vi "moc_energia_sygn_okr.vi"() -> ()   [LabVIEW 2025]
uses:
  <vilib>/measure/NI_MABase.lvlib
panel:
  out "gestosc widmowa mocy":waveform(dbl)(graph)
  out "gestosc widmowa energii":waveform(dbl)(graph)
  out "widmo mocy":waveform(dbl)(graph)
  out "Moc sygn okr":dbl
  out "energia":dbl
  out "spektrum ampl":waveform(dbl)(graph)
  out "As2":dbl[](array[numeric])
  out "As":dbl[](array[numeric])
  out "sygnal":waveform(dbl)(graph)
  out "df":dbl
  in  "offset":dbl format="%0.2p"
  in  "signal type":T1(ring)
  in  "frequency":dbl=10.0 format="%0.2p"
  in  "amplitude":dbl=1.0 format="%0.2p"
  in  "phase":dbl format="%.2p"
  in  "square wave duty cycle (%)":dbl=50.0 format="%0.2f"
  in  "sampling info":cluster{"Fs":dbl, "#s":dbl}={"Fs"=1000.0, "#s"=1000.0} {"Fs" format="%.2p"}
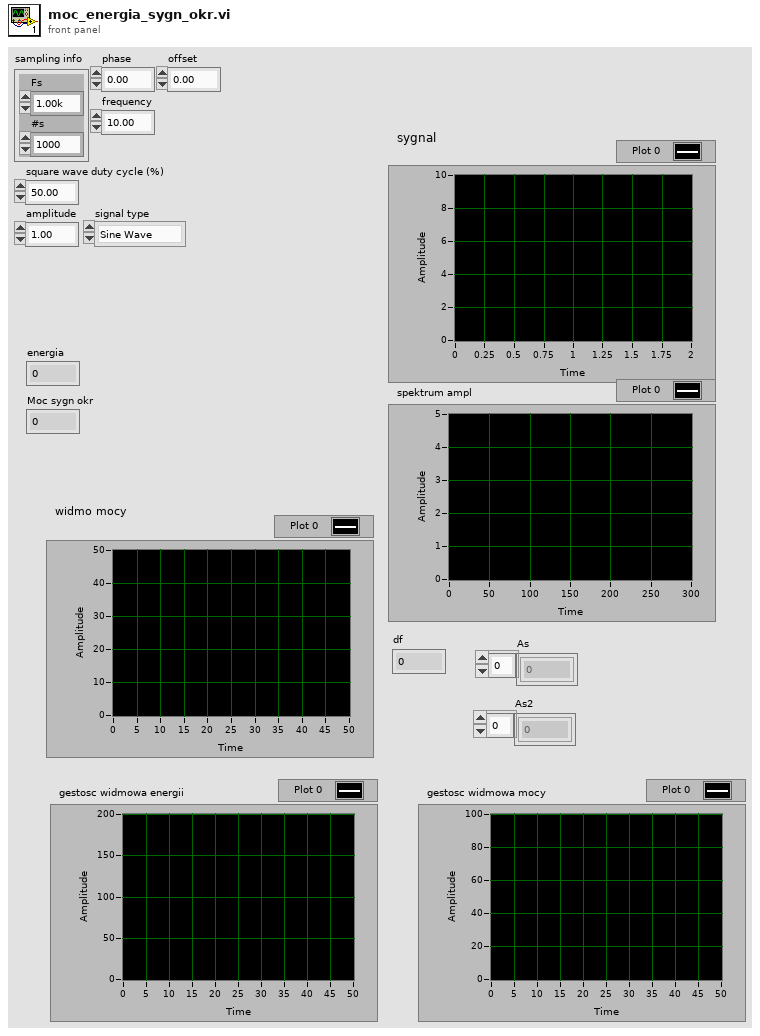
[diagram p1: front panel]
types:
  T1 = enum16{"Sine Wave", "Triangle Wave", "Square Wave", "Sawtooth Wave"}
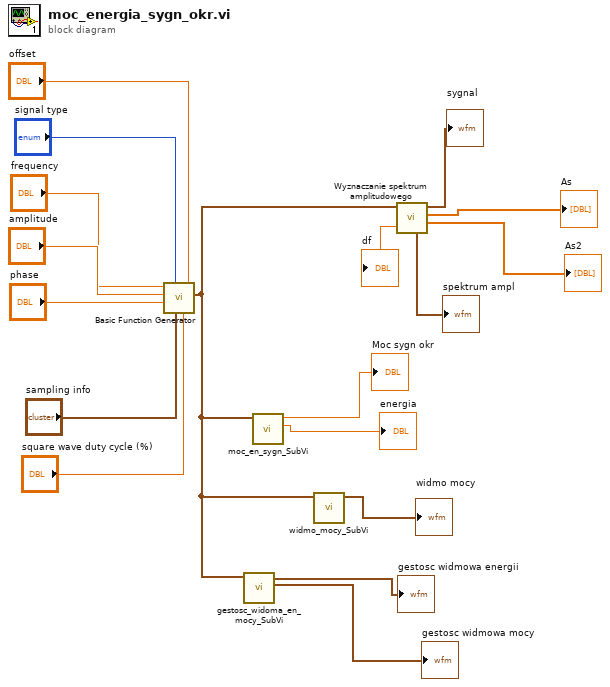
[diagram p0: block diagram]
diagram:
  n1 = call <vilib>:"Basic Function Generator.vi"("offset"="offset", "square wave duty cycle (%)"="square wave duty cycle (%)", "sampling info"="sampling info", "signal type"="signal type", "phase"="phase", "amplitude"="amplitude", "frequency"="frequency") -> ("signal out"=w3:waveform(dbl))  [unwired: 2 in, 2 out]
  n2 = call "gestosc_widoma_en_mocy_SubVi.vi"("signal in"=w3) -> ("gestosc widmowa mocy"=→"gestosc widmowa mocy":waveform(dbl), "gestosc widmowa energii"=→"gestosc widmowa energii":waveform(dbl))  [unwired: 9 in]
  n3 = call "moc_en_sygn_SubVi.vi"("signal in"=w3) -> ("energia"=→"energia":dbl, "Moc sygn okr"=→"Moc sygn okr":dbl)  [unwired: 9 in]
  n4 = call "widmo_mocy_SubVi.vi"("signal in"=w3) -> ("widmo mocy"=→"widmo mocy":waveform(dbl))  [unwired: 10 in]
  n5 = call "Wyznaczanie spektrum amplitudowego.vi"("signal in"=w3) -> ("As2"=→"As2":dbl[], "As"=→"As":dbl[], "Waveform Graph"=→"sygnal":waveform(dbl), "Waveform"=→"spektrum ampl":waveform(dbl), "df"=→"df":dbl)  [unwired: 5 in, 1 out]
